vi "syslog sequential status.vi"(8 "error in (no error)":errorcluster, 9 "sequential tags?":bool, 10 "shared memory name":string, 11 "shared memory runtime in":refnum<class "Shared Memory runtime.lvclass">) -> (0 "error out":errorcluster, 3 "shared memory runtime out":refnum<class "Shared Memory runtime.lvclass">)   [LabVIEW 2013, in "Shared Memory runtime.lvclass"]
uses:
  Shared Memory runtime.lvclass
  <vilib>/NI/Syslog Wrapper - Linux/write syslog.vi
  <vilib>/Utility/LVClass/Get LV Class Name.vi
  <vilib>/NI/Tag Bus Module Framework/runtime/TBM module execution interface.lvclass
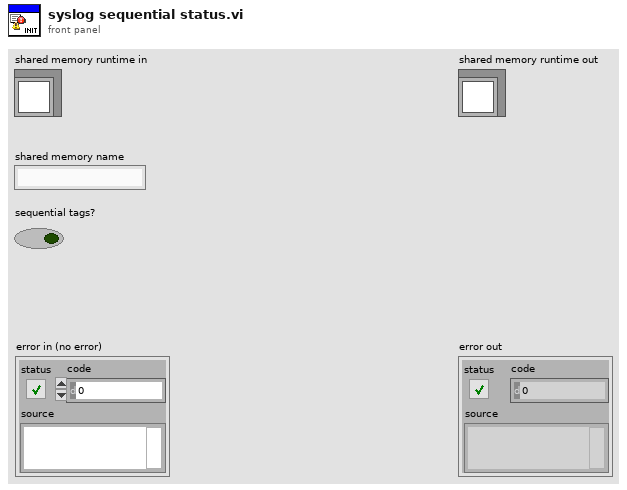
[diagram p1: front panel]
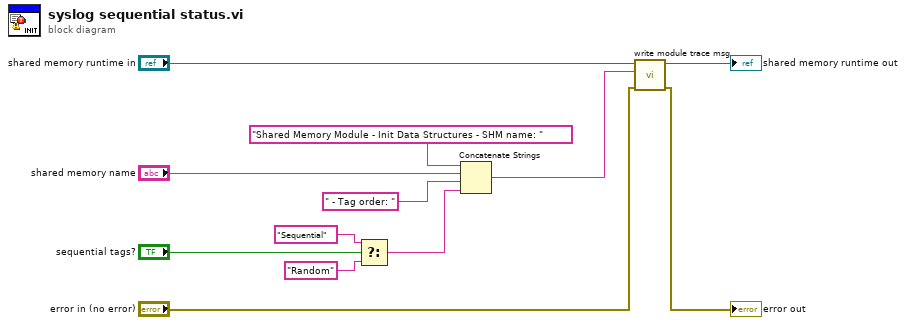
[diagram p0: block diagram]
diagram:
  n1 = Select(t="Sequential", s="sequential tags?", f="Random") -> (s? t:f=w4:string)
  n2 = Concatenate Strings("Shared Memory Module - Init Data Structures - SHM name: ", "shared memory name", " - Tag order: ", w4) -> (w1:string)
  n3 = call <vilib>:"write module trace msg.vi"("error in (no error)"="error in (no error)", "message"=w1, "module in"="shared memory runtime in") -> ("error out"=→"error out":errorcluster, "module out"=→"shared memory runtime out":refnum<class "Shared Memory runtime.lvclass">)  [unwired: 7 in]
